vi "Message Class.vi"(8 "error in (no error)":errorcluster, 11 "Message":refnum<class "MSG.lvclass">) -> (0 "error out":errorcluster, 2 "Message Class":string, 3 "Message":refnum<class "MSG.lvclass">)   [LabVIEW 2011, in "Messenging.lvlib" / "MSG.lvclass"]
uses:
  MSG.lvclass
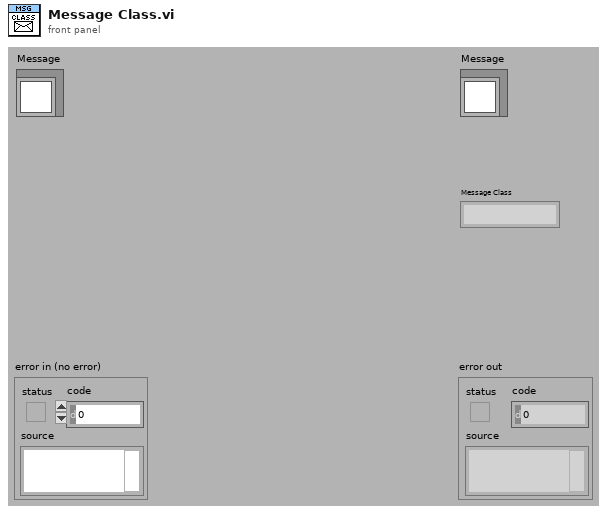
[diagram p1: front panel]
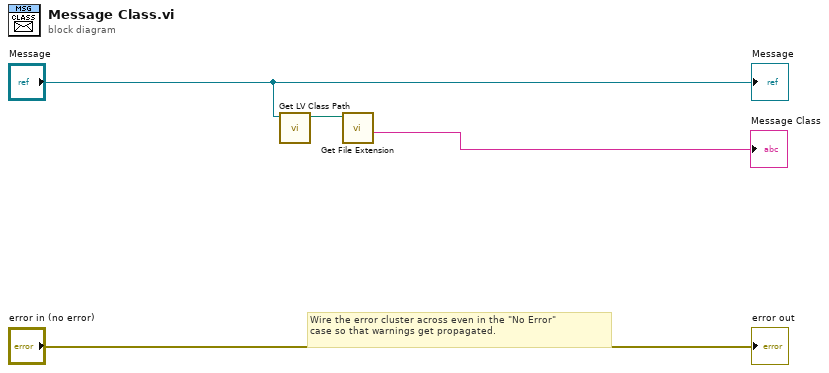
[diagram p0: block diagram]
diagram:
  # "Wire the error cluster across even in the \"No Error\"\ncase so that warnings get propagated."
  n1 = call <vilib>:"Get LV Class Path.vi"("object"="Message") -> ("class path"=w2:path)  [unwired: 1 in, 9 out]
  n2 = call <vilib>:"Get File Extension.vi"("file"=w2) -> ("filename without extension"=→"Message Class":string)  [unwired: 1 in, 9 out]
  "error out" <- "error in (no error)"
  "Message" <- "Message"
